vi "RT sender&receiver.vi"() -> ()   [LabVIEW 2017]
panel:
  out "Number Received from Host":i32
  in  "stop":bool
  out "Sent String to Host":string
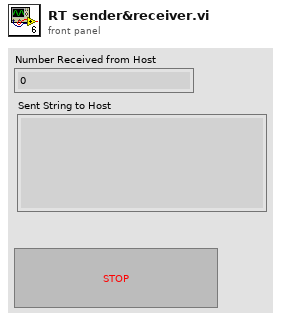
[diagram p1: front panel]
types:
  T1 = cluster{"Xpos":dbl, "Ypos":dbl, "Fx":dbl, "Fy":dbl}
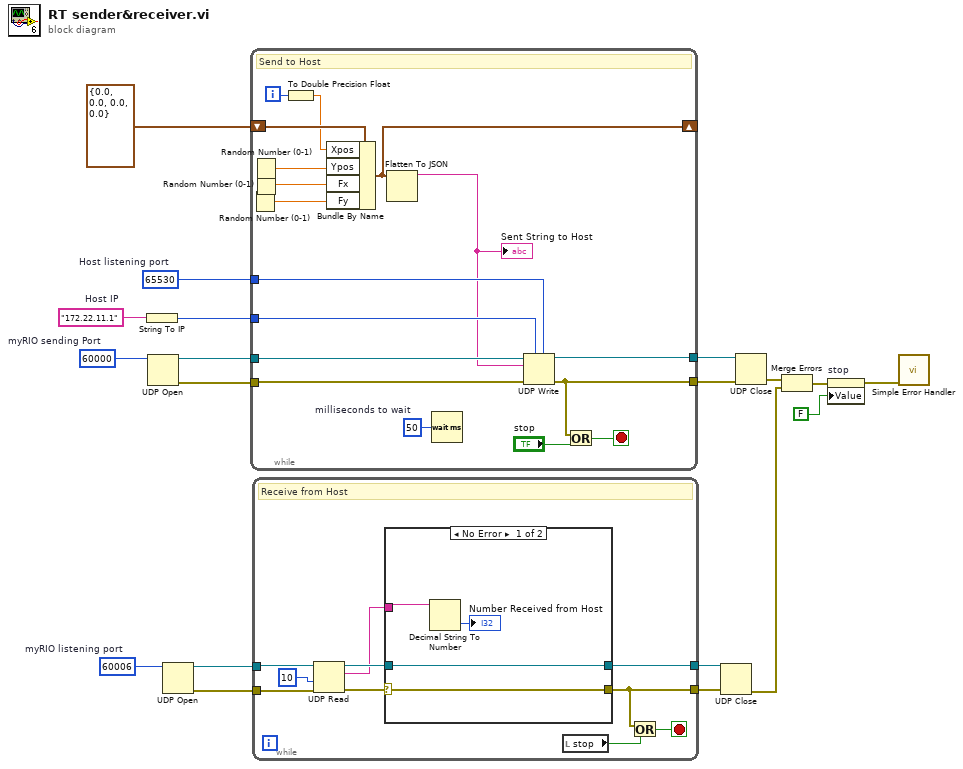
[diagram p0: block diagram]
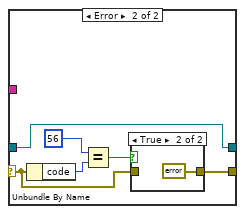
[diagram p2: hidden frame]
diagram:
  w9 = u16 60006  # myRIO listening port
  w14 = u16 65530  # Host listening port
  w16 = "172.22.11.1"  # Host IP
  w19 = u16 60000  # myRIO sending Port
  n1 = String To IP(1:w16) -> (0:w15:u32)
  n2 = UDP Open(11:w19) -> (port=w17:refnum<k16>, 0:w18:errorcluster)  [unwired: 4 in, 1 out]
  n3 = UDP Open(11:w9) -> (port=w11:refnum<k16>, 0:w10:errorcluster)  [unwired: 4 in, 1 out]
  n4 = while {
    tunnel: w18 -> [w34]
    tunnel: w17 -> [w35]
    tunnel: w15 -> [w33]
    tunnel: w14 -> [w32]
    tunnel: [w31] -> w13
    tunnel: [w29] -> w12
    shift-right: [w22] -> _
    shift-left: T1 {"Xpos"=0.0, "Ypos"=0.0, "Fx"=0.0, "Fy"=0.0} -> [w27]
    i -> [w25]
    stop <- w30 stop-if-true
    w36 = u32 50  # milliseconds to wait
    # "Send to Host"
    n5 = Random Number (0-1)() -> (number: 0 to 1=w20:dbl)
    n6 = Random Number (0-1)() -> (number: 0 to 1=w26:dbl)
    n7 = Random Number (0-1)() -> (number: 0 to 1=w21:dbl)
    n8 = To Double Precision Float(number=w25) -> (double precision float=w24:dbl)
    n9 = Bundle By Name(cluster=w27, "Xpos"=w24, "Ypos"=w26, "Fx"=w21, "Fy"=w20) -> (w22:T1)
    n10 = Flatten To JSON(anything=w22) -> (JSON string=w23:string)  [unwired: 2 in, 1 out]
    "Sent String to Host" <- w23
    n11 = Wait (ms)(milliseconds to wait=w36) -> ()  [unwired: 1 out]
    n12 = UDP Write(address=w33, port or service name=w32, connection ID=w35, data in=w23, 8:w34) -> (error out=w29:errorcluster, 3:w31:refnum<k16>)  [unwired: 1 in]
    n13 = Or(x=w29, y="stop") -> (x .or. y?=w30:bool)
  }
  n14 = while {
    tunnel: w11 -> [w46]
    tunnel: w10 -> [w45]
    tunnel: [w38] -> w8
    tunnel: [w40] -> w7
    stop <- w39 stop-if-true
    # "Receive from Host"
    n15 = UDP Read(connection ID=w46, timeout ms (25000)=10, 8:w45) -> (data out=w41:string, error out=w43:errorcluster, 3:w42:refnum<k16>)  [unwired: 1 in, 2 out]
    n16 = case shown="No Error" w43 {
      selector: w43 -> [w50 w52]
      tunnel: w42 -> [w49 w51]
      tunnel: w41 -> [w48 _]
      tunnel: [w50 w53] -> w38
      tunnel: [w49 w51] -> w40
      frame No Error {
        n17 = Decimal String To Number(string=w48) -> (number=→"Number Received from Host":i32)  [unwired: 2 in, 1 out]
      }
      frame Error {
        n18 = Unbundle By Name(w52) -> ("code"=w56:i32)
        n19 = Equal?(x=56, y=w56) -> (x = y?=w54:bool)
        n20 = case shown="True" w54 {
          tunnel: [w57 errorcluster {"status"=FALSE, "code"=0, "source"=""} ("error constant")] -> w53
          tunnel: w52 -> [w57 _]
          frame False {
          }
          frame True {
          }
        }
      }
    }
    n21 = local read "stop"() -> (w37:bool)
    n22 = Or(x=w38, y=w37) -> (x .or. y?=w39:bool)
  }
  n23 = UDP Close(connection ID=w7, 8:w8) -> (error out=w3:errorcluster)  [unwired: 1 out]
  n24 = UDP Close(connection ID=w13, 8:w12) -> (error out=w6:errorcluster)  [unwired: 1 out]
  n25 = Merge Errors(w6, w3) -> (w5:errorcluster)
  n26 = property on="stop" class="Bool (strict)"(error in=w5, "Value"=FALSE ("stop")) -> (error out=w4:errorcluster)  [unwired: 1 in, 1 out]
  n27 = call <vilib>:"Simple Error Handler.vi"("error in (no error)"=w4) -> ()  [unwired: 4 in, 5 out]
